vi "ParseReading.vi"(11 "Data":u16[](array[numeric]) format="%04x") -> (2 "Voltage":dbl, 3 "Freq":dbl)   [LabVIEW 2021]
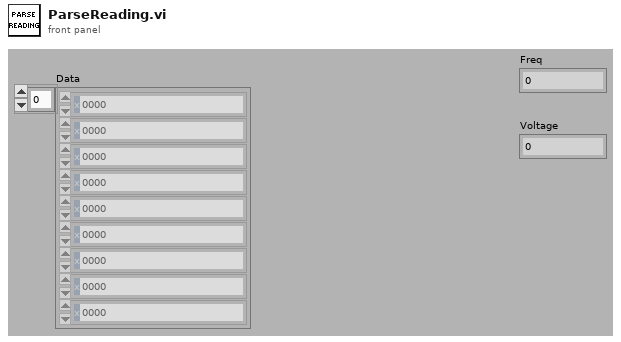
[diagram p1: front panel]
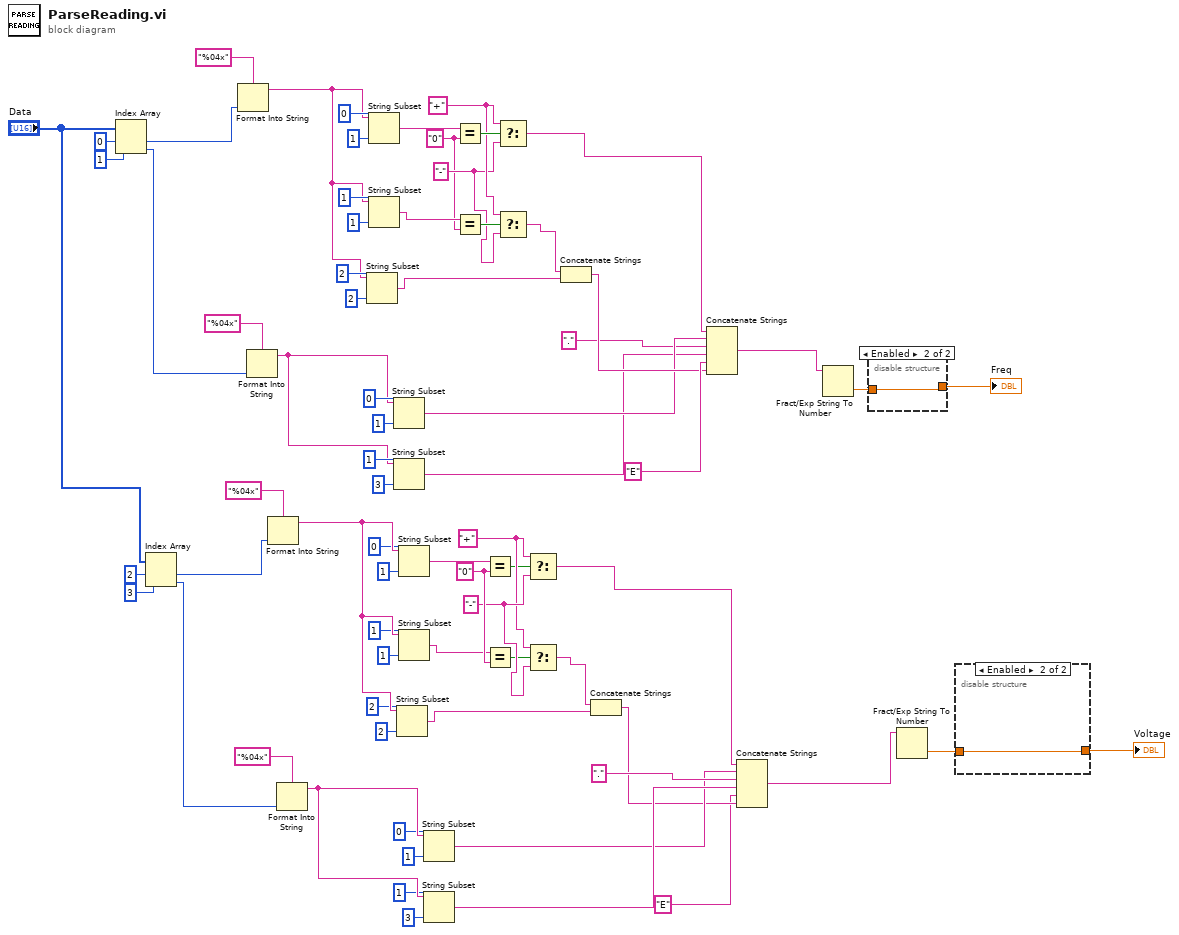
[diagram p0: block diagram]
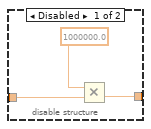
[diagram p2: hidden frame]
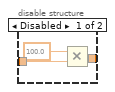
[diagram p3: hidden frame]
diagram:
  w29 = "-" ("y")
  w28 = "+" ("y")
  w30 = "0" ("y")
  w48 = "-" ("y")
  w49 = "+" ("y")
  w47 = "0" ("y")
  n1 = Index Array(array="Data", index #1=0 ("index"), index #2=1 ("index")) -> (element #1=w71:u16, element #2=w55:u16)
  n2 = Index Array(array="Data", index #1=2 ("index"), index #2=3 ("index")) -> (element #1=w8:u16, element #2=w24:u16)
  n3 = Format Into String(format string="%04x", w71) -> (resulting string=w59:string)  [unwired: 2 in, 1 out]
  n4 = Format Into String(format string="%04x", w55) -> (resulting string=w39:string)  [unwired: 2 in, 1 out]
  n5 = Format Into String(format string="%04x", w8) -> (resulting string=w20:string)  [unwired: 2 in, 1 out]
  n6 = Format Into String(format string="%04x", w24) -> (resulting string=w38:string)  [unwired: 2 in, 1 out]
  n7 = String Subset(string=w59, offset (0)=2, length (rest)=2 ("length (rest)")) -> (substring=w57:string)
  n8 = String Subset(string=w59, offset (0)=0, length (rest)=1 ("length (rest)")) -> (substring=w67:string)
  n9 = String Subset(string=w59, offset (0)=1, length (rest)=1 ("length (rest)")) -> (substring=w62:string)
  n10 = String Subset(string=w39, offset (0)=0, length (rest)=1 ("length (rest)")) -> (substring=w44:string)
  n11 = String Subset(string=w39, offset (0)=1, length (rest)=3 ("length (rest)")) -> (substring=w40:string)
  n12 = String Subset(string=w20, offset (0)=2, length (rest)=2 ("length (rest)")) -> (substring=w22:string)
  n13 = String Subset(string=w20, offset (0)=0, length (rest)=1 ("length (rest)")) -> (substring=w12:string)
  n14 = String Subset(string=w20, offset (0)=1, length (rest)=1 ("length (rest)")) -> (substring=w17:string)
  n15 = String Subset(string=w38, offset (0)=0, length (rest)=1 ("length (rest)")) -> (substring=w33:string)
  n16 = String Subset(string=w38, offset (0)=1, length (rest)=3 ("length (rest)")) -> (substring=w37:string)
  n17 = Equal?(x=w67, y=w47) -> (x = y?=w66:bool)
  n18 = Equal?(x=w62, y=w47) -> (x = y?=w63:bool)
  n19 = Equal?(x=w12, y=w30) -> (x = y?=w13:bool)
  n20 = Equal?(x=w17, y=w30) -> (x = y?=w16:bool)
  n21 = Select(t=w49, s=w66, f=w48) -> (s? t:f=w54:string)
  n22 = Select(t=w49, s=w63, f=w48) -> (s? t:f=w58:string)
  n23 = Select(t=w28, s=w13, f=w29) -> (s? t:f=w25:string)
  n24 = Select(t=w28, s=w16, f=w29) -> (s? t:f=w21:string)
  n25 = Concatenate Strings(w58, w57) -> (w52:string)
  n26 = Concatenate Strings(w21, w22) -> (w27:string)
  n27 = Concatenate Strings(w54, w44, "." ("string"), w40, "E" ("string"), w52) -> (w51:string)
  n28 = Concatenate Strings(w25, w33, "." ("string"), w37, "E" ("string"), w27) -> (w3:string)
  n29 = Fract/Exp String To Number(string=w51) -> (number=w50:dbl)  [unwired: 3 in, 1 out]
  n30 = disable-structure shown="Enabled" {
    disable-tunnel: w50 -> [w76 w77]
    disable-tunnel: [w75 w77] -> w1
    frame Disabled {
      n31 = Multiply(x=100.0, y=w76) -> (x*y=w75:dbl)
    }
    frame Enabled {
    }
  }
  "Freq" <- w1
  n32 = Fract/Exp String To Number(string=w3) -> (number=w4:dbl)  [unwired: 3 in, 1 out]
  n33 = disable-structure shown="Enabled" {
    disable-tunnel: w4 -> [w80 w81]
    disable-tunnel: [w79 w81] -> w2
    frame Disabled {
      n34 = Multiply(x=1000000.0, y=w80) -> (x*y=w79:dbl)
    }
    frame Enabled {
    }
  }
  "Voltage" <- w2
